vi "S.K.Y Controller Global.vi"() -> ()   [LabVIEW 2019]
panel:
  in  "Right Slider":dbl
  in  "POV":dbl[](array[numeric])
  in  "Left Slider":dbl
  in  "X Axis":dbl
  in  "Rotate":dbl
  in  "Y Axis":dbl
  out "Scroll up":bool
  out "Back Right":bool
  out "Front Button":bool
  out "Scroll down":bool
  out "Back left":bool
  out "Bottom D":bool
  out "Bottom C":bool
  out "Bottom A":bool
  out "Bottom B":bool
  out "Top Right":bool
  out "Top Left":bool
  out "Bottom Right":bool
  out "Bottom Left":bool
  out "Trigger":bool
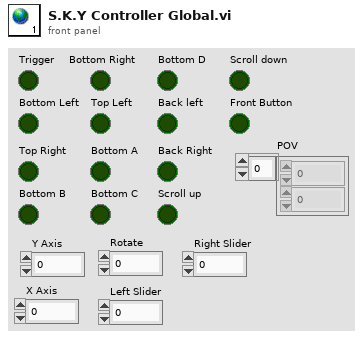
[diagram p1: front panel]
diagram:
